vi "Get Hi Times Wind Speed V.vi"(8 "error in (no error)":errorcluster, 11 "DateTimeHiWindSpeed":T1) -> (0 "error out":errorcluster, 2 "function return":i16, 3 "DateTimeHiWindSpeed out":T1)   [LabVIEW 2009, in "VantagePro.lvlib"]
doc: "DllAccess short int _stdcall GetHiTimesWindSpeed_V (DateTime* DateTimeHiWindSpeed);"
uses:
  VantagePro.lvlib
  <userlib>/VantagePro/VantagePro.dll
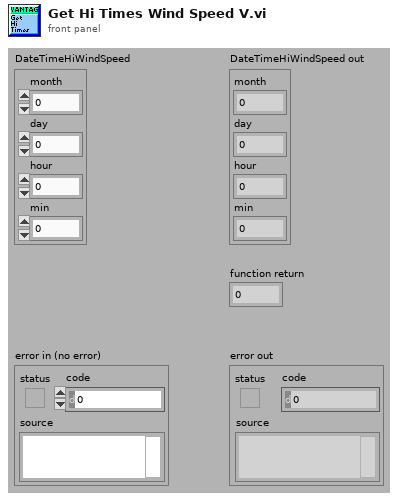
[diagram p1: front panel]
types:
  T1 = cluster{"month":i16, "day":i16, "hour":i16, "min":i16}
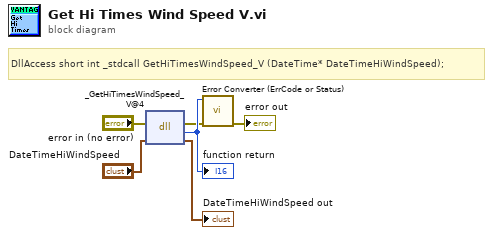
[diagram p0: block diagram]
diagram:
  # "DllAccess short int _stdcall GetHiTimesWindSpeed_V (DateTime* DateTimeHiWindSpeed);"
  n1 = dll-call lib="C:/Program Files/National Instruments/LabVIEW 2010/user.lib/VantagePro/VantagePro.*" fn="_GetHiTimesWindSpeed_V@4"(error in="error in (no error)", "DateTimeHiWindSpeed"="DateTimeHiWindSpeed") -> (error out=w2:errorcluster, w6:i16, "DateTimeHiWindSpeed"=→"DateTimeHiWindSpeed out":T1)  [unwired: 2 in, 1 out]
  "function return" <- w6
  n2 = call "Error Converter (ErrCode or Status).vi"("error in (no error)"=w2, "error code"=w6) -> ("error out"=→"error out":errorcluster)  [unwired: 9 in]
